vi "Flipping the Ramans.vi"(0 "Folder Name":string, 1 "Name of File":string, 2 "Timepoints":dbl[](array[numeric]), 3 "Vx array":dbl[](array[numeric]), 4 "Vy array":dbl[](array[numeric])) -> ()   [LabVIEW 2014]
uses:
  <vilib>/Utility/file.llb/Write Delimited Spreadsheet (DBL).vi
  <vilib>/Utility/file.llb/Read Delimited Spreadsheet (DBL).vi
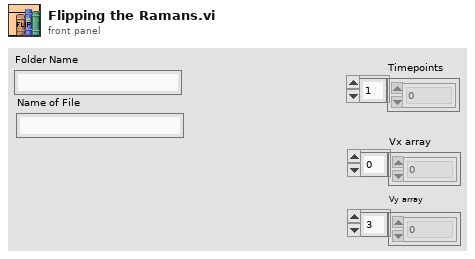
[diagram p1: front panel]
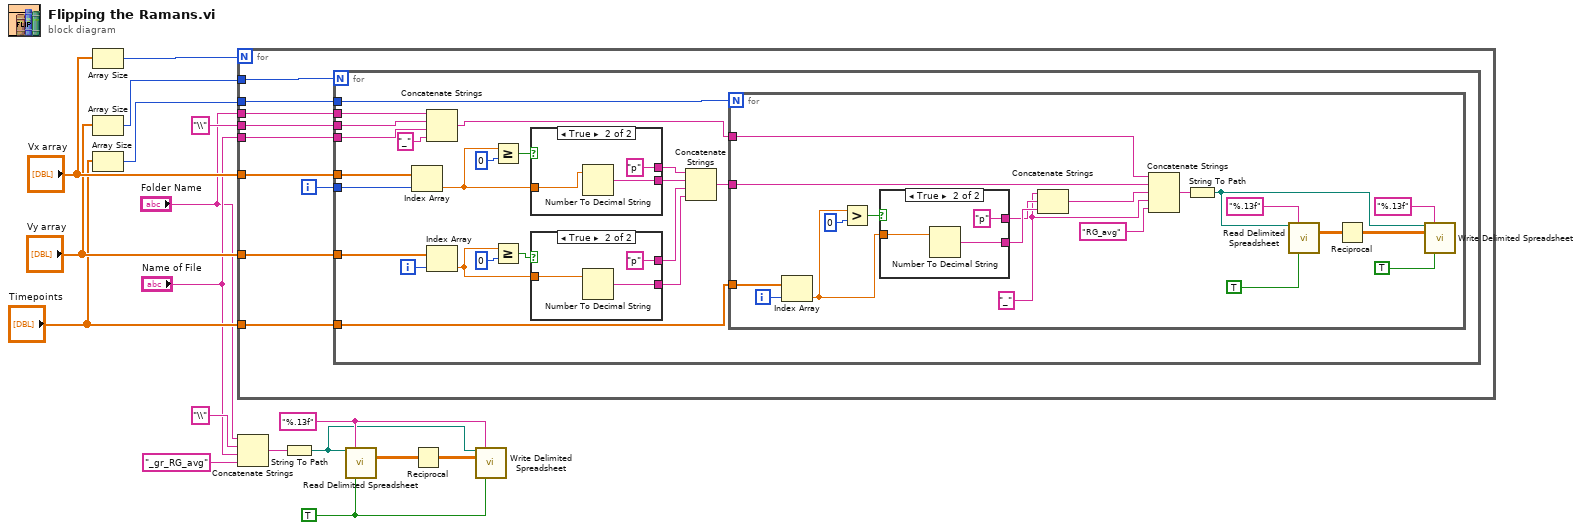
[diagram p0: block diagram]
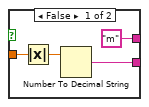
[diagram p2: hidden frame]
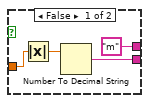
[diagram p3: hidden frame]
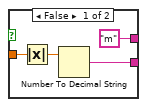
[diagram p4: hidden frame]
diagram:
  w3 = "%.13f" ("format (%.3f)")
  w2 = TRUE ("transpose? (F)")
  n1 = Array Size(array="Vx array") -> (size(s)=w16:i32)
  n2 = Array Size(array="Vy array") -> (size(s)=w15:i32)
  n3 = Array Size(array="Timepoints") -> (size(s)=w14:i32)
  n4 = for {
    N: w16 -> [_]
    tunnel: "Name of File" -> [w26]
    tunnel: "\\" -> [w25]
    tunnel: "Folder Name" -> [w24]
    tunnel: w15 -> [w23]
    tunnel: w14 -> [w22]
    tunnel: "Vx array" -> [w21]
    tunnel: "Vy array" -> [w19]
    tunnel: "Timepoints" -> [w18]
    i -> [w20]
    n5 = for {
      N: w23 -> [_]
      tunnel: w26 -> [w27]
      tunnel: w25 -> [w28]
      tunnel: w24 -> [w48]
      tunnel: w22 -> [w47]
      tunnel: w21 -> [w43]
      tunnel: w20 -> [w44]
      tunnel: w19 -> [w38]
      tunnel: w18 -> [w32]
      i -> [w37]
      n6 = Index Array(array=w43, index=w44) -> (element=w42:dbl)
      n7 = Concatenate Strings(w48, w28, w27, "_") -> (w30:string)
      n8 = Index Array(array=w38, index=w37) -> (element=w39:dbl)
      n9 = Greater Or Equal?(x=w42, y=0) -> (x >= y?=w45:bool)
      n10 = Greater Or Equal?(x=w39, y=0) -> (x >= y?=w41:bool)
      n11 = case shown="True" w45 {
        tunnel: ["m" "p"] -> w36
        tunnel: w42 -> [w58 w60]
        tunnel: [w56 w61] -> w35
        frame False {
          n12 = Absolute Value(x=w58) -> (abs(x)=w57:dbl)
          n13 = Number To Decimal String(number=w57) -> (decimal integer string=w56:string)  [unwired: 1 in]
        }
        frame True {
          n14 = Number To Decimal String(number=w60) -> (decimal integer string=w61:string)  [unwired: 1 in]
        }
      }
      n15 = case shown="True" w41 {
        tunnel: ["m" "p"] -> w34
        tunnel: w39 -> [w51 w53]
        tunnel: [w49 w54] -> w33
        frame False {
          n16 = Absolute Value(x=w51) -> (abs(x)=w50:dbl)
          n17 = Number To Decimal String(number=w50) -> (decimal integer string=w49:string)  [unwired: 1 in]
        }
        frame True {
          n18 = Number To Decimal String(number=w53) -> (decimal integer string=w54:string)  [unwired: 1 in]
        }
      }
      n19 = Concatenate Strings(w36, w35, w34, w33) -> (w29:string)
      n20 = for {
        N: w47 -> [_]
        tunnel: w32 -> [w79]
        tunnel: w30 -> [w70]
        tunnel: w29 -> [w69]
        i -> [w78]
        w68 = "_"
        n21 = Index Array(array=w79, index=w78) -> (element=w81:dbl)
        n22 = Greater?(x=w81, y=0) -> (0:w80:bool)
        n23 = case shown="True" w80 {
          tunnel: ["m" "p"] -> w76
          tunnel: w81 -> [w85 w87]
          tunnel: [w83 w88] -> w77
          frame False {
            n24 = Absolute Value(x=w85) -> (abs(x)=w84:dbl)
            n25 = Number To Decimal String(number=w84) -> (decimal integer string=w83:string)  [unwired: 1 in]
          }
          frame True {
            n26 = Number To Decimal String(number=w87) -> (decimal integer string=w88:string)  [unwired: 1 in]
          }
        }
        n27 = Concatenate Strings(w68, w76, w77) -> (w64:string)
        n28 = Concatenate Strings(w70, w69, w64, w68, "RG_avg") -> (w72:string)
        n29 = String To Path(string=w72) -> (path=w63:path)
        n30 = call-poly <vilib>:"Read Delimited Spreadsheet.vi"("file path (dialog if empty)"=w63, "format (%.3f)"="%.13f", "transpose? (F)"=TRUE) -> ("all rows"=w66:dbl[][])  [unwired: 7 in, 5 out]
        n31 = Reciprocal(x=w66) -> (1/x=w65:dbl[][])
        n32 = call-poly <vilib>:"Write Delimited Spreadsheet.vi"("file path (dialog if empty)"=w63, "format (%.3f)"="%.13f", "2D data"=w65, "transpose? (F)"=TRUE) -> ()  [unwired: 10 in, 2 out]
      }
    }
  }
  n33 = Concatenate Strings("Folder Name", "\\" ("string"), "Name of File", "_gr_RG_avg" ("string")) -> (w7:string)
  n34 = String To Path(string=w7) -> (path=w1:path)
  n35 = call-poly <vilib>:"Read Delimited Spreadsheet.vi"("file path (dialog if empty)"=w1, "format (%.3f)"=w3, "transpose? (F)"=w2) -> ("all rows"=w5:dbl[][])  [unwired: 7 in, 5 out]
  n36 = Reciprocal(x=w5) -> (1/x=w4:dbl[][])
  n37 = call-poly <vilib>:"Write Delimited Spreadsheet.vi"("file path (dialog if empty)"=w1, "format (%.3f)"=w3, "2D data"=w4, "transpose? (F)"=w2) -> ()  [unwired: 10 in, 2 out]
